vi "Listen_wait.vi"(8 "error in (no error)":errorcluster, 11 "Socket.TCP in":refnum<class "Socket.TCP.lvclass">) -> (0 "error out":errorcluster, 3 "Socket.TCP out":refnum<class "Socket.TCP.lvclass">)   [LabVIEW 2014, in "Socket.lvlib" / "Socket.TCP.lvclass"]
doc: "Waits for an accepted TCP network connection. Saves the remote_address and remote_port of the accepted connection when one arrives."
uses:
  Socket.TCP.lvclass
  Socket.TCP.lvclass/Socket.TCP.ctl
  Socket.Base/Socket.Base.lvclass/Socket.Base.ctl
  Accessors/Read listener_refnum.vi
  Socket.Base/Accessors/Read timeout.vi
  Accessors/Write listener_refnum.vi
  Accessors/Write remote_address .vi
  Accessors/Write remote_port .vi
  Accessors/Write tcp _refnum.vi
  Socket.Base/Accessors/Write connected.vi
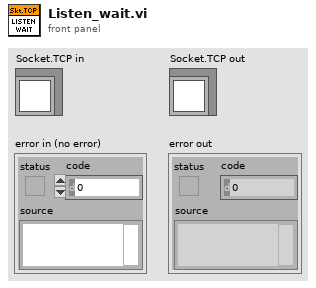
[diagram p1: front panel]
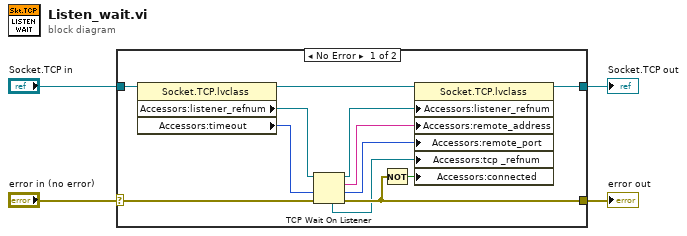
[diagram p0: block diagram]
diagram:
  n1 = case shown="No Error" "error in (no error)" {
    selector: "error in (no error)" -> [w15 w18]
    tunnel: [w9 w18] -> w3
    tunnel: [w11 w17] -> w1
    tunnel: "Socket.TCP in" -> [w16 w17]
    frame No Error {
      n2 = property class="Socket.TCP.lvclass"(reference=w16) -> (reference out=w14:refnum<class "Socket.TCP.lvclass">, "Accessors:listener_refnum"=w13:refnum<k5>, "Accessors:timeout"=w12:i32)  [unwired: 1 in, 1 out]
      n3 = TCP Wait On Listener(8:w15, 9:w12, 11:w13) -> (0:w9:errorcluster, 1:w6:u16, 2:w7:string, 3:w8:refnum<k5>, 4:w5:refnum<k5>)  [unwired: 1 in]
      n4 = Not(x=w9) -> (.not. x?=w10:bool)
      n5 = property class="Socket.TCP.lvclass"(reference=w14, "Accessors:listener_refnum"=w8, "Accessors:remote_address "=w7, "Accessors:remote_port "=w6, "Accessors:tcp _refnum"=w5, "Accessors:connected"=w10) -> (reference out=w11:refnum<class "Socket.TCP.lvclass">)  [unwired: 1 in, 1 out]
    }
    frame Error {
    }
  }
  "error out" <- w3
  "Socket.TCP out" <- w1
